vi "module.Layouts.Save.vi"(7 "modules":T1[][](array[typedef]), 10 "Columns":u8=1 min=1 max=10 step=1, 11 "Rows":u8=1 min=1 max=10 step=1) -> (2 "spreadsheet string":string)   [LabVIEW 2020]
uses:
  _controls/element.ctl
  <vilib>/Utility/file.llb/Write Delimited Spreadsheet (I64).vi
panel:
  out "error out":errorcluster
  in  "error in":errorcluster
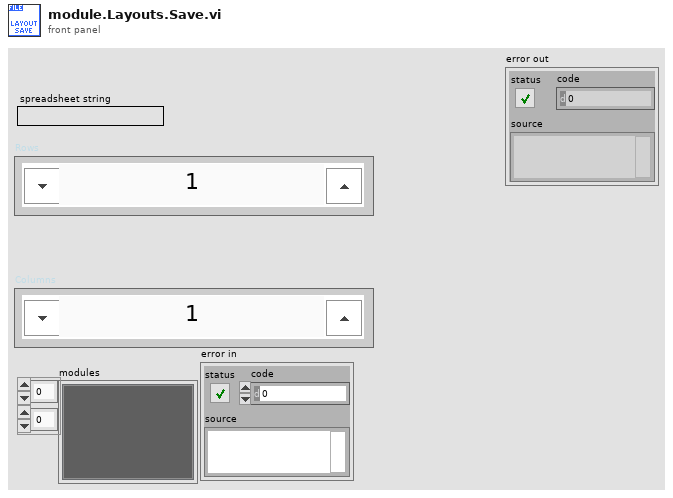
[diagram p1: front panel]
types:
  T1 = typedef "element.ctl" = cluster{"Color Box":u32, "label":string}
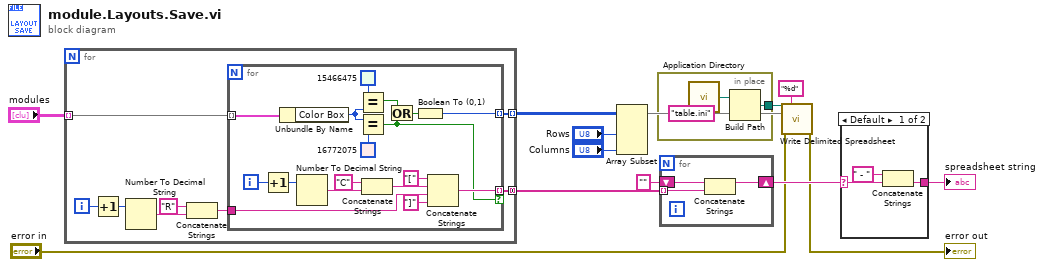
[diagram p0: block diagram]
diagram:
  n1 = for {
    tunnel: "modules" -> [w21] mode=indexing
    tunnel: [w20] -> w9 mode=indexing
    tunnel: [w19] -> w7 mode=concatenating
    i -> [w15]
    n2 = Increment(x=w15) -> (x+1=w17:i32)
    n3 = Number To Decimal String(number=w17) -> (decimal integer string=w18:string)  [unwired: 1 in]
    n4 = Concatenate Strings("R" ("string"), w18) -> (w14:string)
    n5 = for {
      tunnel: w21 -> [w38] mode=indexing
      tunnel: [w36] -> w20 mode=indexing
      tunnel: w14 -> [w31]
      tunnel: [w28] -> w19 mode=indexing if=w27
      i -> [w23]
      n6 = Increment(x=w23) -> (x+1=w26:i32)
      n7 = Unbundle By Name(w38) -> ("Color Box"=w35:u32)
      n8 = Number To Decimal String(number=w26) -> (decimal integer string=w25:string)  [unwired: 1 in]
      n9 = Equal?(x=u32 15466475, y=w35) -> (x = y?=w32:bool)
      n10 = Equal?(x=w35, y=u32 16772075) -> (x = y?=w27:bool)
      n11 = Concatenate Strings("C" ("string"), w25) -> (w22:string)
      n12 = Or(x=w32, y=w27) -> (x .or. y?=w33:bool)
      n13 = Boolean To (0,1)(Boolean=w33) -> (0, 1=w36:i16)
      n14 = Concatenate Strings("[" ("string"), w22, w31, "]" ("string")) -> (w28:string)
    }
  }
  n15 = Array Subset(array=w9, length (row)="Rows", length (col)="Columns") -> (w12:i16[][])  [unwired: 2 in]
  n16 = in-place {
    in-place-border: [w40] -> w11
    n17 = call <vilib>:"Application Directory.vi"() -> ("Application Directory"=w41:path)
    n18 = Build Path(base path=w41, name or relative path="table.ini" ("format (%d)")) -> (appended path=w40:path)
  }
  n19 = for {
    tunnel: w7 -> [w44] mode=indexing
    shift-right: [w43] -> w5
    shift-left: "" -> [w42]
    n20 = Concatenate Strings(w42, w44) -> (w43:string)
  }
  n21 = call-poly <vilib>:"Write Delimited Spreadsheet.vi"("file path (dialog if empty)"=w11, "format (%d)"="%d", "2D data"=w12, "error in (no error)"="error in") -> ("error out"=→"error out":errorcluster)  [unwired: 10 in, 1 out]
  n22 = case shown="Default" w5 {
    selector: w5 -> [w46 w48]
    tunnel: [w47 w48] -> w4
    frame Default {
      n23 = Concatenate Strings(" - " ("string"), w46) -> (w47:string)
    }
    frame "" {
    }
  }
  "spreadsheet string" <- w4
